vi "Set Dynamic Parameters.vi"(8 "error in (no error)":errorcluster, 10 "dynamic parameters":T2={"mass"=0.0, "gear ratio"=0.0, "motor inertia"=0.0, "center of gravity"=[], "viscous friction"=0.0, "positive coulomb friction"=0.0, "negative coulomb friction"=0.0, "inertia matrix"=[[0.0, 0.0, 0.0], [0.0, 0.0, 0.0], [0.0, 0.0, 0.0]]}, 11 "Link in":refnum<class "Link.lvclass">) -> (0 "error out":errorcluster, 3 "Link out":refnum<class "Link.lvclass">)   [LabVIEW 2013, in "Link.lvclass"]
uses:
  Link.lvclass
  <vilib>/Analysis/Matrix/Datatypes/RealMatrix.ctl
  Link.lvclass/Link.ctl
  <vilib>/Analysis/Matrix/NI_Matrix.lvlib
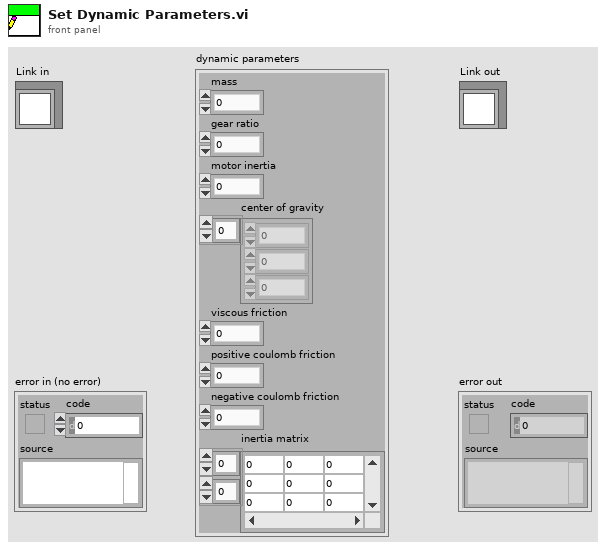
[diagram p1: front panel]
types:
  T1 = typedef "NI_Matrix.lvlib/RealMatrix.ctl" = dbl[][]
  T2 = cluster{"mass":dbl, "gear ratio":dbl, "motor inertia":dbl, "center of gravity":dbl[], "viscous friction":dbl, "positive coulomb friction":dbl, "negative coulomb friction":dbl, "inertia matrix":T1}
  T3 = cluster{"positive coulomb friction":dbl, "negative coulomb friction":dbl}
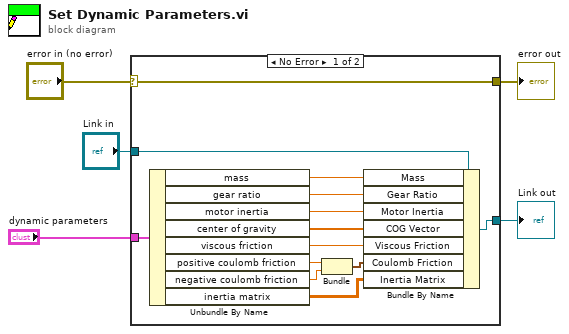
[diagram p0: block diagram]
diagram:
  n1 = case shown="No Error" "error in (no error)" {
    selector: "error in (no error)" -> [w18 w19]
    tunnel: [w18 w19] -> w4
    tunnel: [w16 w20] -> w2
    tunnel: "Link in" -> [w17 w20]
    tunnel: "dynamic parameters" -> [w15 _]
    frame No Error {
      n2 = Unbundle By Name(w15) -> ("mass"=w12:dbl, "gear ratio"=w9:dbl, "motor inertia"=w10:dbl, "center of gravity"=w11:dbl[], "viscous friction"=w8:dbl, "positive coulomb friction"=w14:dbl, "negative coulomb friction"=w13:dbl, "inertia matrix"=w6:T1)
      n3 = Bundle("positive coulomb friction"=w14, "negative coulomb friction"=w13) -> (w7:T3)  [unwired: 1 in]
      n4 = Bundle By Name(cluster=w17, "Mass"=w12, "Gear Ratio"=w9, "Motor Inertia"=w10, "COG Vector"=w11, "Viscous Friction"=w8, "Coulomb Friction"=w7, "Inertia Matrix"=w6) -> (w16:refnum<class "Link.lvclass">)
    }
    frame Error {
    }
  }
  "error out" <- w4
  "Link out" <- w2
